vi "Msg.vi"(7 "jettl in":refnum<class "jettl.lvclass">, 11 "Set Panel State Msg Strategy in":refnum<class "Set Panel State Msg Strategy.lvclass">) -> (5 "jettl out":refnum<class "jettl.lvclass">)   [LabVIEW 2021, in "Set Panel State Msg Strategy.lvlib" / "Set Panel State Msg Strategy.lvclass"]
uses:
  Set Panel State Msg Strategy.lvclass
  jettl/jettl/jettl.lvclass
  Set Panel State/Set Panel State.lvclass
  Set Panel State Msg Strategy.lvclass/Set Panel State Msg Strategy.ctl
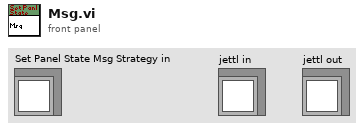
[diagram p1: front panel]
types:
  T1 = enum32{"Invalid", "Standard", "Closed", "Hidden", "Minimized", "Maximized"}
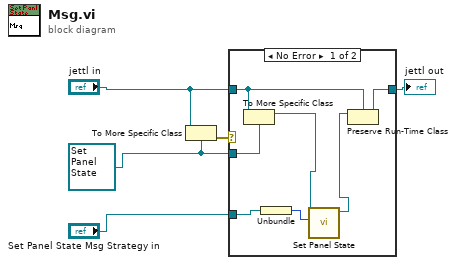
[diagram p0: block diagram]
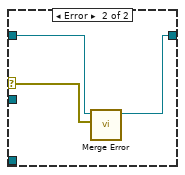
[diagram p2: hidden frame]
diagram:
  w2 = refnum<class "Set Panel State.lvclass"> refnum ("Panel Open Msg Strategy.lvlib:Panel Open.lvclass")
  n1 = To More Specific Class(target class=w2, reference="jettl in") -> (error out=w5:errorcluster)  [unwired: 1 in, 1 out]
  n2 = case shown="No Error" w5 {
    selector: w5 -> [_ w15]
    tunnel: [w10 w13] -> w3
    tunnel: "jettl in" -> [w11 w14]
    tunnel: w2 -> [w12 _]
    tunnel: "Set Panel State Msg Strategy in" -> [w7 _]
    frame No Error {
      n3 = To More Specific Class(target class=w12, reference=w11) -> (specific class reference=w9:refnum<class "Set Panel State.lvclass">)  [unwired: 1 in, 1 out]
      n4 = Unbundle "Unbundle"(w7) -> (w6:T1)
      n5 = call-dynamic "Set Panel State.vi"("Front Panel Window:State"=w6, "Set Panel State in"=w9) -> ("Set Panel State out"=w8:refnum<class "Set Panel State.lvclass">)  [unwired: 9 in]
      n6 = Preserve Run-Time Class(object in=w8, 2:w11) -> (object out=w10:refnum<class "jettl.lvclass">)  [unwired: 1 in, 1 out]
    }
    frame Error {
      n7 = call-dynamic "Merge Error.vi"("Error"=w15, "Merge Error in"=w14) -> ("Merge Error out"=w13:refnum<class "jettl.lvclass">)  [unwired: 9 in]
    }
  }
  "jettl out" <- w3
